vi "Login.vi"() -> ()   [LabVIEW 2019, in "User Lib.lvlib"]
uses:
  User Lib.lvlib
  database.lvlib
panel:
  out "Username Ref":refnum<vi>
  in  "Cancel":bool
  in  "OK":bool
  in  "Password":string
  in  "Username":string
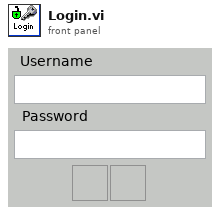
[diagram p1: front panel]
types:
  T1 = cluster{i32, "date/time string":string, "date/time string":string, string}
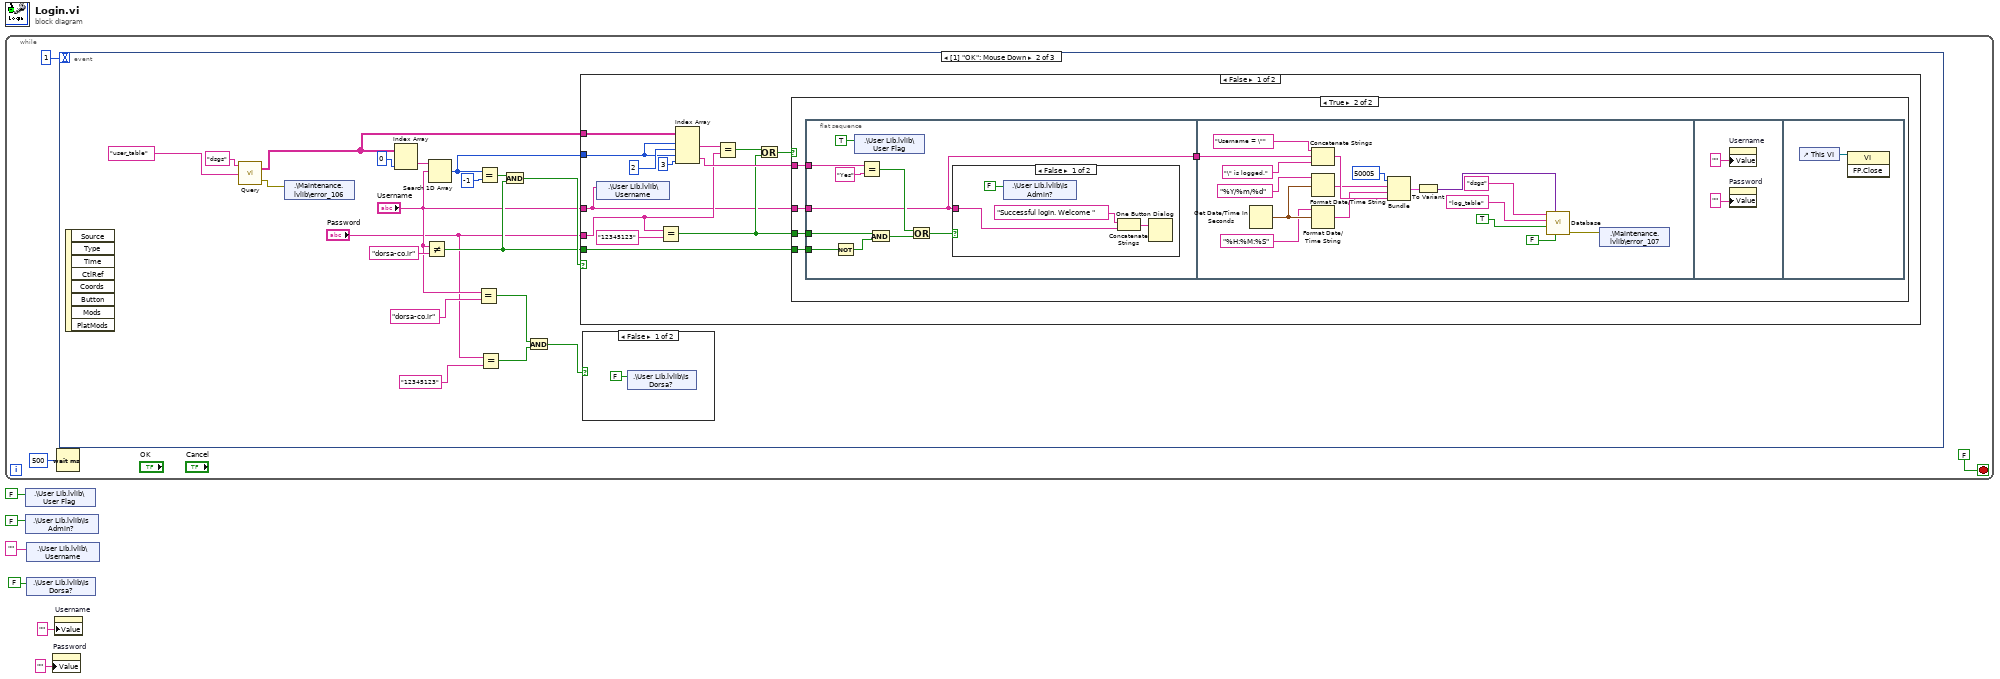
[diagram p0: block diagram]
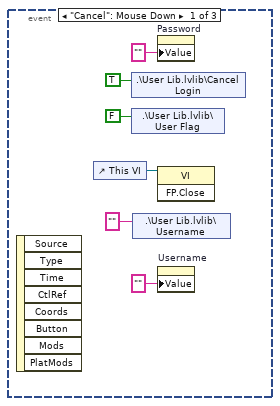
[diagram p2: hidden frame]
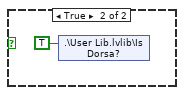
[diagram p3: hidden frame]
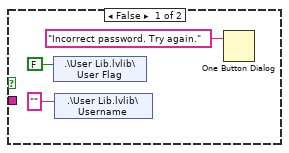
[diagram p4: hidden frame]
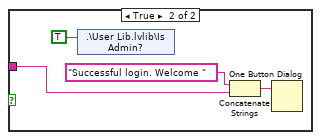
[diagram p5: hidden frame]
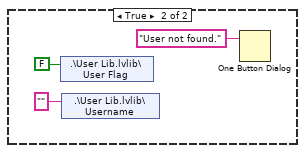
[diagram p6: hidden frame]
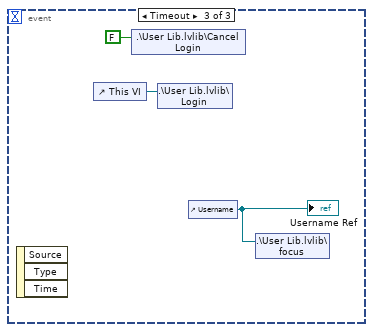
[diagram p7: hidden frame]
diagram:
  n1 = while {
    stop <- FALSE stop-if-true
    n2 = Wait (ms)(milliseconds to wait=u32 500) -> ()  [unwired: 1 out]
    n3 = event shown="[1] \"OK\": Mouse Down" {
      selector: _ -> [_ _ _]
      dyn-events: _ -> [_ _ _]
      timeout: 1 -> [_ _ _]
      event "Cancel": Mouse Down {
        n4 = event-data() -> ()  [unwired: 1 in, 8 out]
        n5 = control-ref of="This VI"() -> (w15:refnum<vi>)
        n6 = shared-variable ".\\User Lib.lvlib\\Cancel Login"(TRUE ("Login Boolean")) -> ()  [unwired: 1 in, 1 out]
        n7 = shared-variable ".\\User Lib.lvlib\\User Flag"(FALSE ("User Flag")) -> ()  [unwired: 1 in, 1 out]
        n8 = shared-variable ".\\User Lib.lvlib\\Username"("" ("Username")) -> ()  [unwired: 1 in, 1 out]
        n9 = property on="Password" class="Str"("Value"="" ("Password")) -> ()  [unwired: 2 in, 2 out]
        n10 = invoke class="VI" method="FP.Close"(reference=w15) -> ()  [unwired: 2 in, 3 out]
        n11 = property on="Username" class="Str"("Value"="" ("Username")) -> ()  [unwired: 2 in, 2 out]
      }
      event "OK": Mouse Down {
        n12 = event-data() -> ()  [unwired: 1 in, 8 out]
        n13 = call "Query.vi"("Table Name"="user_table", "Connection Name"="dsgs") -> ("Error out"=w23:errorcluster, "data"=w28:string[][])  [unwired: 2 in]
        n14 = shared-variable ".\\Maintenance.lvlib\\error_106"(w23) -> ()  [unwired: 1 in, 1 out]
        n15 = Index Array(array=w28, index (col)=0 ("disabled index (col)")) -> (element=w33:string[])  [unwired: 1 in]
        n16 = Not Equal?(x="Username", y="dorsa-co.ir") -> (x != y?=w24:bool)
        n17 = Search 1D Array(1D array=w33, element="Username") -> (index of element=w31:i32)  [unwired: 1 in]
        n18 = Equal?(x="Username", y="dorsa-co.ir") -> (x = y?=w18:bool)
        n19 = Equal?(x=w31, y=-1) -> (x = y?=w26:bool)
        n20 = Equal?(x="Password", y="12345123") -> (x = y?=w17:bool)
        n21 = And(x=w26, y=w24) -> (x .and. y?=w25:bool)
        n22 = And(x=w18, y=w17) -> (x .and. y?=w16:bool)
        n23 = case shown="False" w25 {
          tunnel: w28 -> [w49 _]
          tunnel: w31 -> [w45 _]
          tunnel: "Password" -> [w40 _]
          tunnel: "Username" -> [w37 _]
          tunnel: w24 -> [w39 _]
          frame False {
            n24 = shared-variable ".\\User Lib.lvlib\\Username"(w37) -> ()  [unwired: 1 in, 1 out]
            n25 = Equal?(x=w40, y="12345123" ("x")) -> (x = y?=w38:bool)
            n26 = Index Array(array=w49, index (row) #1=w45, index (col) #1=2 ("disabled index (col)"), index (row) #2=w45, index (col) #2=3 ("index (col)")) -> (element #1=w47:string, element #2=w44:string)
            n27 = Equal?(x=w47, y=w40) -> (x = y?=w43:bool)
            n28 = Or(x=w43, y=w38) -> (x .or. y?=w42:bool)
            n29 = case shown="True" w42 {
              tunnel: w44 -> [_ w57]
              tunnel: w39 -> [_ w56]
              tunnel: w38 -> [_ w55]
              tunnel: w37 -> [_ w54]
              frame False {
                n30 = shared-variable ".\\User Lib.lvlib\\User Flag"(FALSE ("User Flag")) -> ()  [unwired: 1 in, 1 out]
                n31 = shared-variable ".\\User Lib.lvlib\\Username"("" ("Username")) -> ()  [unwired: 1 in, 1 out]
                n32 = One Button Dialog(message="Incorrect password. Try again.") -> ()  [unwired: 1 in, 1 out]
              }
              frame True {
                n33 = flat-sequence {
                  tunnel: w57 -> [w65]
                  tunnel: w56 -> [w60]
                  tunnel: w55 -> [w64]
                  tunnel: w54 -> [w58]
                  tunnel: [w58] -> w53
                  tunnel: w53 -> [w77]
                  frame #0 {
                    n34 = Not(x=w60) -> (.not. x?=w59:bool)
                    n35 = shared-variable ".\\User Lib.lvlib\\User Flag"(TRUE) -> ()  [unwired: 1 in, 1 out]
                    n36 = Equal?(x=w65, y="Yes") -> (x = y?=w63:bool)
                    n37 = And(x=w64, y=w59) -> (x .and. y?=w62:bool)
                    n38 = Or(x=w63, y=w62) -> (x .or. y?=w61:bool)
                    n39 = case shown="False" w61 {
                      tunnel: w58 -> [w69 w73]
                      frame False {
                        n40 = shared-variable ".\\User Lib.lvlib\\Is Admin?"(FALSE ("Is Admin?")) -> ()  [unwired: 1 in, 1 out]
                        n41 = Concatenate Strings("Successful login. Welcome " ("message"), w69) -> (w68:string)
                        n42 = One Button Dialog(message=w68) -> ()  [unwired: 1 in, 1 out]
                      }
                      frame True {
                        n43 = shared-variable ".\\User Lib.lvlib\\Is Admin?"(TRUE ("Is Admin?")) -> ()  [unwired: 1 in, 1 out]
                        n44 = Concatenate Strings("Successful login. Welcome " ("message"), w73) -> (w72:string)
                        n45 = One Button Dialog(message=w72) -> ()  [unwired: 1 in, 1 out]
                      }
                    }
                  }
                  frame #1 {
                    n46 = Get Date/Time In Seconds() -> (seconds since 1Jan1904=w91:timestamp)
                    n47 = Concatenate Strings("Username = \"" ("string"), w77, "\" is logged." ("string")) -> (w92:string)
                    n48 = Format Date/Time String(time format string (%c)="%Y/%m/%d", seconds (now)=w91) -> (date/time string=w90:string)  [unwired: 1 in]
                    n49 = Format Date/Time String(time format string (%c)="%H:%M:%S", seconds (now)=w91) -> (date/time string=w89:string)  [unwired: 1 in]
                    n50 = Bundle(50005, "date/time string"=w90, "date/time string"=w89, w92) -> (w88:T1)  [unwired: 1 in]
                    n51 = To Variant(anything=w88) -> (Variant=w87:variant)
                    n52 = call "Database.vi"("Delete row?"=FALSE, "Data"=w87, "Auto Increment ID?"=TRUE, "Table"="log_table" ("table"), "Connection"="dsgs" ("table")) -> ("Error out"=w76:errorcluster)  [unwired: 6 in]
                    n53 = shared-variable ".\\Maintenance.lvlib\\error_107"(w76) -> ()  [unwired: 1 in, 1 out]
                  }
                  frame #2 {
                    n54 = property on="Username" class="Str"("Value"="" ("Username")) -> ()  [unwired: 2 in, 2 out]
                    n55 = property on="Password" class="Str"("Value"="" ("Password")) -> ()  [unwired: 2 in, 2 out]
                  }
                  frame #3 {
                    n56 = control-ref of="This VI"() -> (w95:refnum<vi>)
                    n57 = invoke class="VI" method="FP.Close"(reference=w95) -> ()  [unwired: 2 in, 3 out]
                  }
                }
              }
            }
          }
          frame True {
            n58 = shared-variable ".\\User Lib.lvlib\\User Flag"(FALSE ("User Flag")) -> ()  [unwired: 1 in, 1 out]
            n59 = shared-variable ".\\User Lib.lvlib\\Username"("" ("Username")) -> ()  [unwired: 1 in, 1 out]
            n60 = One Button Dialog(message="User not found.") -> ()  [unwired: 1 in, 1 out]
          }
        }
        n61 = case shown="False" w16 {
          frame False {
            n62 = shared-variable ".\\User Lib.lvlib\\Is Dorsa?"(FALSE ("Is Dorsa?")) -> ()  [unwired: 1 in, 1 out]
          }
          frame True {
            n63 = shared-variable ".\\User Lib.lvlib\\Is Dorsa?"(TRUE ("Is Dorsa?")) -> ()  [unwired: 1 in, 1 out]
          }
        }
      }
      event Timeout {
        n64 = event-data() -> ()  [unwired: 1 in, 3 out]
        n65 = control-ref of="This VI"() -> (w101:refnum<vi>)
        n66 = shared-variable ".\\User Lib.lvlib\\Cancel Login"(FALSE ("Login Boolean")) -> ()  [unwired: 1 in, 1 out]
        n67 = shared-variable ".\\User Lib.lvlib\\Login"(w101) -> ()  [unwired: 1 in, 1 out]
        n68 = control-ref of="Username"() -> (w99:refnum<vi>)
        "Username Ref" <- w99
        n69 = shared-variable ".\\User Lib.lvlib\\focus"(w99) -> ()  [unwired: 1 in, 1 out]
      }
    }
  }
  n70 = shared-variable ".\\User Lib.lvlib\\User Flag"(FALSE ("User Flag")) -> ()  [unwired: 1 in, 1 out]
  n71 = shared-variable ".\\User Lib.lvlib\\Is Admin?"(FALSE ("Is Admin?")) -> ()  [unwired: 1 in, 1 out]
  n72 = shared-variable ".\\User Lib.lvlib\\Username"("" ("Username")) -> ()  [unwired: 1 in, 1 out]
  n73 = shared-variable ".\\User Lib.lvlib\\Is Dorsa?"(FALSE ("Is Dorsa?")) -> ()  [unwired: 1 in, 1 out]
  n74 = property on="Password" class="Str"("Value"="" ("Password")) -> ()  [unwired: 2 in, 2 out]
  n75 = property on="Username" class="Str"("Value"="" ("Username")) -> ()  [unwired: 2 in, 2 out]
